vi "Make Child and Move.vi"(7 "Process Name":string, 9 "Name of Parent Panel":string, 10 "New Center Coords":T1, 11 "VI in":refnum<vi>) -> ()   [LabVIEW 2018]
doc: "Make the VI Ref a Child Window of the named Parent Window and move to new coordinates."
uses:
  <vilib>/Utility/miscctls.llb/LVPoint32TypeDef.ctl
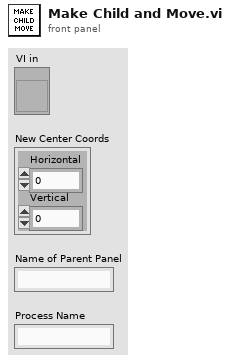
[diagram p1: front panel]
types:
  T1 = typedef "LVPoint32TypeDef.ctl" = cluster{"Horizontal":i32, "Vertical":i32}
  T2 = enum32{"Invalid", "Standard", "Closed", "Hidden", "Minimized", "Maximized"}
  T3 = typedef "LVRectTypeDef.ctl" = cluster{"Left":i16, "Top":i16, "Right":i16, "Bottom":i16}
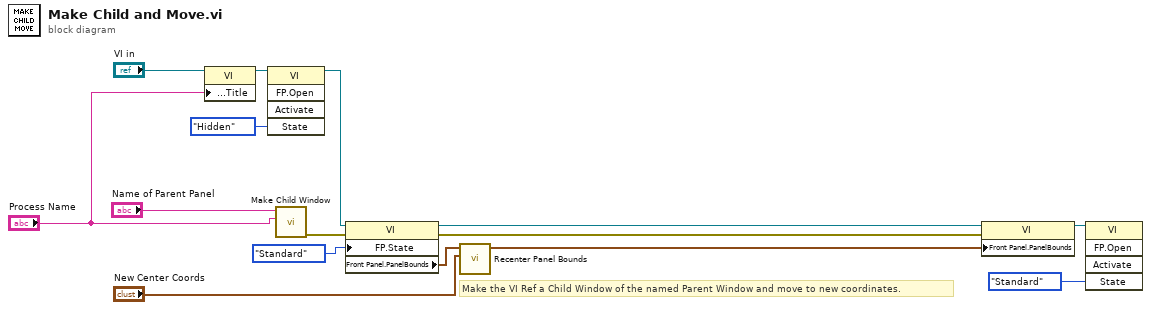
[diagram p0: block diagram]
diagram:
  # "Make the VI Ref a Child Window of the named Parent Window and move to new coordinates."
  n1 = property class="VI"(reference="VI in", "Front Panel.Title"="Process Name") -> (reference out=w2:refnum<vi>)  [unwired: 1 in, 1 out]
  n2 = invoke class="VI" method="FP.Open"(reference=w2, "State"=T2."Hidden") -> (reference out=w14:refnum<vi>)  [unwired: 3 in, 4 out]
  n3 = call "Make Child Window.vi"("Name of Child Panel"="Process Name", "Name of Parent Panel"="Name of Parent Panel") -> ("error out"=w7:errorcluster)  [unwired: 5 in]
  n4 = property class="VI"(reference=w14, error in=w7, "FP.State"=T2."Standard" ("Front Panel Window:State")) -> (reference out=w6:refnum<vi>, error out=w9:errorcluster, "Front Panel.PanelBounds"=w4:T3)
  n5 = call "Recenter Panel Bounds.vi"("New Center Coords"="New Center Coords", "Front Panel Window:Panel Bounds in"=w4) -> ("Front Panel Window:Panel Bounds out"=w5:T3)  [unwired: 9 in]
  n6 = property class="VI"(reference=w6, error in=w9, "Front Panel.PanelBounds"=w5) -> (reference out=w12:refnum<vi>)  [unwired: 1 out]
  n7 = invoke class="VI" method="FP.Open"(reference=w12, "State"=T2."Standard") -> ()  [unwired: 3 in, 5 out]
